vi "Advanced file handeling.vi"(4 "Data in":T1) -> (1 "File out":T2)   [LabVIEW 2014]
uses:
  <vilib>/Utility/file.llb/Read From Spreadsheet File (DBL).vi
panel:
  out "Delimit":string
  in  "File delimit":u16(ring) items=["Tab", "Comma"]
  out "transposed array":dbl[][](array[numeric])
  in  "Test":bool
  in  "Filename No' format":u16(ring) items=["glucose cuvette (#) 0mm.txt", "glucose cuvette (1) #mm.txt"]
  in  "File okay":bool
  in  "Data layout":u16(ring)=1
  out "Modified scan":string[][](table)
  in  "Crop top":i32 min=0
  out "Scan":string[][](table)
  in  "Crop bottom":dbl min=0.0 format="%#.0g"
  in  "Important thing L":i32[](array[numeric])
  in  "Important thing R":i32[](array[numeric])
  in  "Cancel":bool
  in  "OK":bool
  in  "File style":enum32{"Radio Selection 1", "Radio Selection 2"}(radio)
  in  "Select file":bool
  in  "Path":path
  # "Advanced file handling"
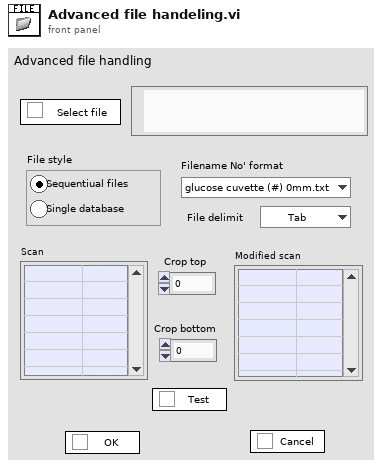
[diagram p1: front panel]
types:
  T1 = cluster{"Path":path, "File style":enum32{"Radio Selection 1", "Radio Selection 2"}, "Filename No' format ":u16, "Data layout":u16, "Crop top":i32, "Crop bottom":dbl, "Important thing R":i32[], "Important thing L":i32[], sgl[][], "Delimit":string}
  T2 = cluster{"Path":path, "File style":enum32{"Radio Selection 1", "Radio Selection 2"}, "Filename No' format ":u16, "Data layout":u16, "Crop top":i32, "Crop bottom":dbl, "Important thing R":i32[], "Important thing L":i32[], sgl[][], "Delimit ":string}
  T3 = enum8{"Enabled", "Disabled", "Disabled and Grayed Out"}
  T4 = cluster{"Path":path, "File style":enum32{"Radio Selection 1", "Radio Selection 2"}, "Filename No' format ":u16, "Data layout":u16, "Crop top":i32, "Crop bottom":dbl, "Important thing R":i32[], "Important thing L":i32[], "transposed array":dbl[][], "Delimit":string}
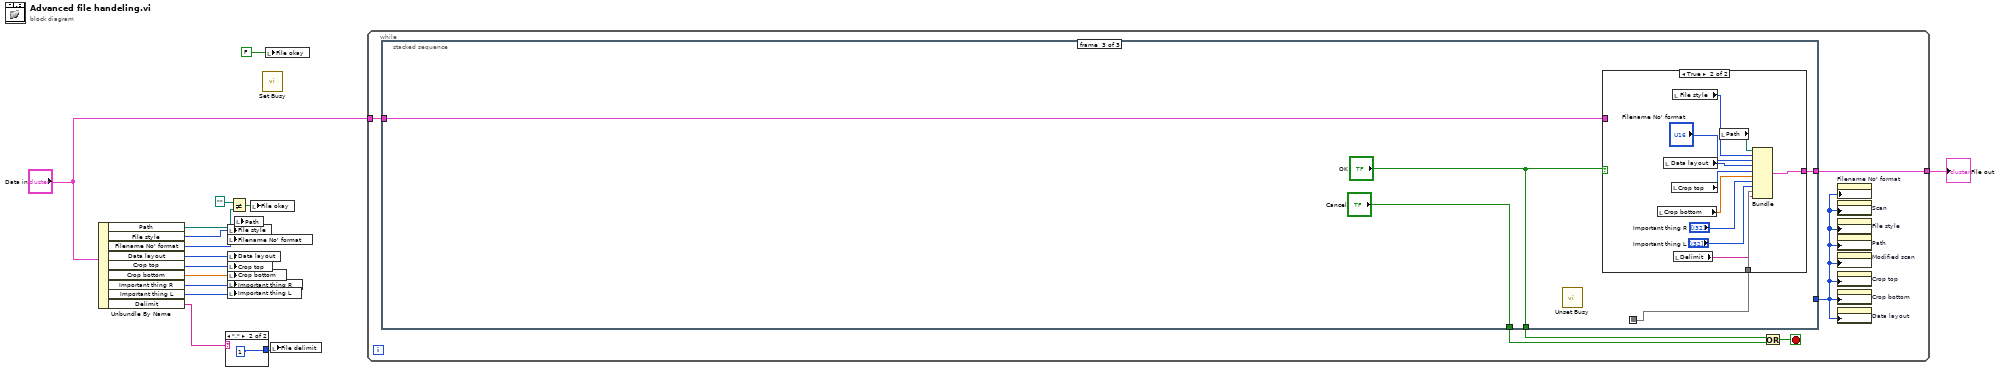
[diagram p0: block diagram]
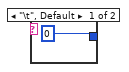
[diagram p2: hidden frame]
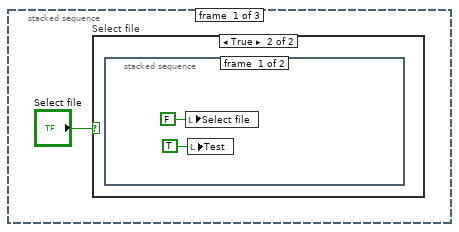
[diagram p3: hidden frame]
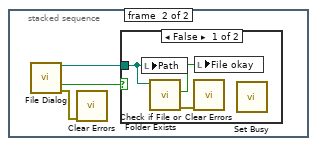
[diagram p5: hidden frame]
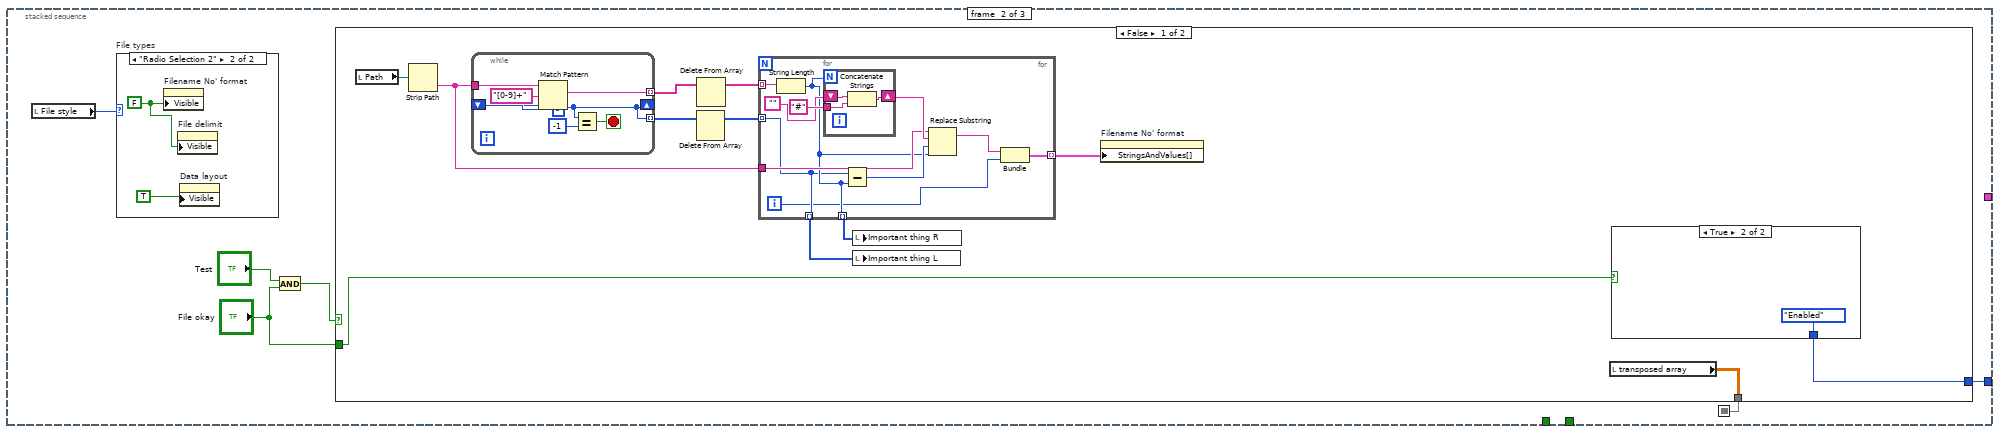
[diagram p7: hidden frame]
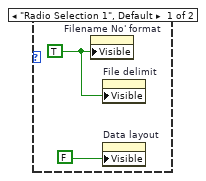
[diagram p8: hidden frame]
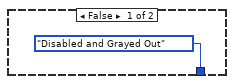
[diagram p9: hidden frame]
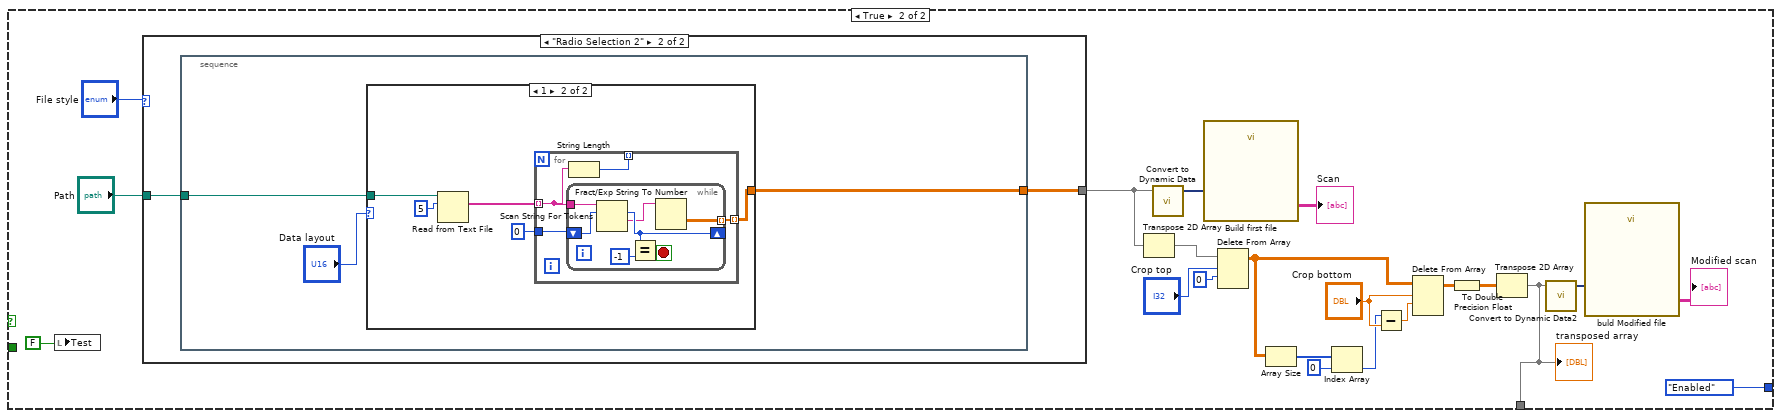
[diagram p10: hidden frame]
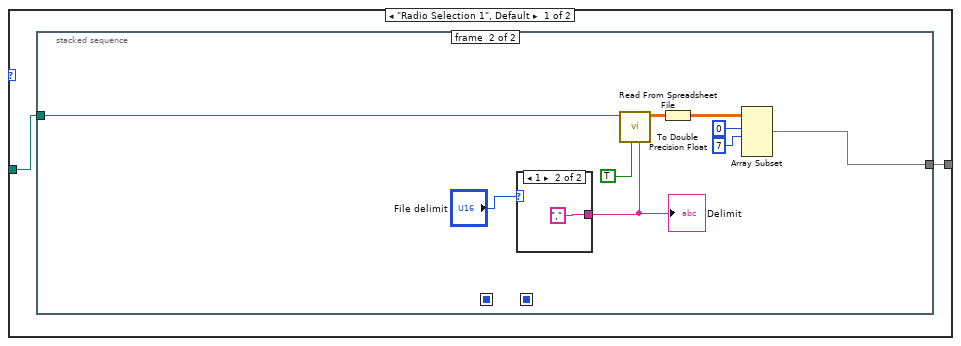
[diagram p11: hidden frame]
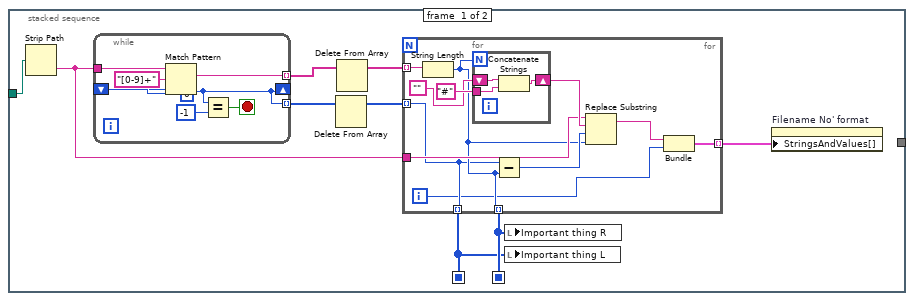
[diagram p12: hidden frame]
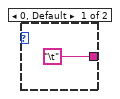
[diagram p13: hidden frame]
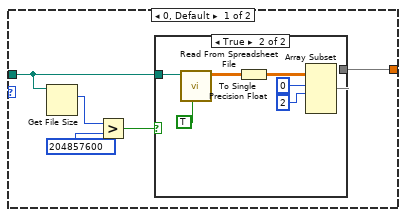
[diagram p14: hidden frame]
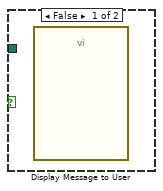
[diagram p15: hidden frame]
diagram:
  n1 = Unbundle By Name("Data in") -> ("Path"=w5:path, "File style"=w11:enum32{"Radio Selection 1", "Radio Selection 2"}, "Filename No' format"=w12:u16, "Data layout"=w10:u16, "Crop top"=w9:i32, "Crop bottom"=w8:dbl, "Important thing R"=w7:i32[], "Important thing L"=w6:i32[], "Delimit"=w2:string)
  n2 = case shown="\",\"" w2 {
    tunnel: [0 1] -> w1
    frame "\t", Default {
    }
    frame "," {
    }
  }
  n3 = local write "File style"(w11) -> ()
  n4 = local write "Filename No' format"(w12) -> ()
  n5 = local write "Data layout"(w10) -> ()
  n6 = local write "Crop top"(w9) -> ()
  n7 = local write "Crop bottom"(w8) -> ()
  n8 = local write "Important thing R"(w7) -> ()
  n9 = local write "Important thing L"(w6) -> ()
  n10 = Not Equal?(x=path "", y=w5) -> (x != y?=w3:bool)
  n11 = local write "Path"(w5) -> ()
  n12 = local write "File okay"(w3) -> ()
  n13 = call <vilib>:"Set Busy.vi"() -> ()  [unwired: 10 in, 2 out]
  n14 = local write "File okay"(FALSE) -> ()
  n15 = local write "File delimit"(w1) -> ()
  n16 = while {
    tunnel: [w20] -> w14
    tunnel: "Data in" -> [w19]
    stop <- w23 stop-if-true
    n17 = stacked-sequence {
      seq-local: [_ w38 _] -> [_ _ w181]
      tunnel: [_ _ "Cancel"] -> w22
      tunnel: [_ _ "OK"] -> w21
      tunnel: [_ _ w178] -> w20
      tunnel: w19 -> [_ _ w177]
      tunnel: [_ w37 _] -> w18
      frame #0 {
        n18 = case "Select file" shown="True" "Select file" {
          frame False {
          }
          frame True {
            n19 = stacked-sequence {
              frame #0 {
                n20 = local write "Select file"(FALSE) -> ()
                n21 = local write "Test"(TRUE) -> ()
              }
              frame #1 {
                n22 = call "File Dialog"() -> ("selected path"=w28:path, "cancelled"=w27:bool, "error out"=w29:errorcluster)  [unwired: 12 in, 1 out]
                n23 = call <vilib>:"Clear Errors.vi"("error in (no error)"=w29) -> ()  [unwired: 5 in, 2 out]
                n24 = case shown="False" w27 {
                  tunnel: w28 -> [w32 _]
                  frame False {
                    n25 = local write "Path"(w32) -> ()
                    n26 = call <vilib>:"Check if File or Folder Exists.vi"("path"=w32) -> ("error out"=w31:errorcluster, "file or folder exists?"=w30:bool)  [unwired: 8 in, 1 out]
                    n27 = call <vilib>:"Clear Errors.vi"("error in (no error)"=w31) -> ()  [unwired: 5 in, 2 out]
                    n28 = local write "File okay"(w30) -> ()
                    n29 = call <vilib>:"Set Busy.vi"() -> ()  [unwired: 10 in, 2 out]
                  }
                  frame True {
                  }
                }
              }
            }
          }
        }
      }
      frame #1 {
        n30 = local read "File style"() -> (w33:enum32{"Radio Selection 1", "Radio Selection 2"})
        n31 = case "File types" shown="\"Radio Selection 2\"" w33 {
          frame "Radio Selection 1", Default {
            w39 = TRUE
            n32 = property on="Filename No' format" class="Ring (strict)"("Visible"=w39) -> ()  [unwired: 2 in, 2 out]
            n33 = property on="File delimit" class="Ring (strict)"("Visible"=w39) -> ()  [unwired: 2 in, 2 out]
            n34 = property on="Data layout" class="Ring (strict)"("Visible"=FALSE) -> ()  [unwired: 2 in, 2 out]
          }
          frame "Radio Selection 2" {
            w41 = FALSE
            n35 = property on="Filename No' format" class="Ring (strict)"("Visible"=w41) -> ()  [unwired: 2 in, 2 out]
            n36 = property on="File delimit" class="Ring (strict)"("Visible"=w41) -> ()  [unwired: 2 in, 2 out]
            n37 = property on="Data layout" class="Ring (strict)"("Visible"=TRUE) -> ()  [unwired: 2 in, 2 out]
          }
        }
        n38 = And(x="Test", y="File okay") -> (x .and. y?=w35:bool)
        n39 = case shown="False" w35 {
          tunnel: [w53 w82] -> w38
          tunnel: [w55 T3."Enabled" ("Disabled")] -> w37
          tunnel: "File okay" -> [w54 _]
          frame False {
            n40 = local read "Path"() -> (w43:path)
            n41 = Strip Path(path=w43) -> (name=w47:string)  [unwired: 1 out]
            n42 = while {
              tunnel: w47 -> [w75]
              shift-right: [w70] -> _
              shift-left: 0 -> [w76]
              tunnel: [w71] -> w50 mode=indexing
              tunnel: [w70] -> w49 mode=indexing
              stop <- w72 stop-if-true
              n43 = Match Pattern(string=w75, regular expression="[0-9]+", offset (0)=w76) -> (match substring=w71:string, offset past match=w70:i32)  [unwired: 2 out]
              n44 = Equal?(x=w70, y=-1) -> (x = y?=w72:bool)
            }
            n45 = Delete From Array(array=w49) -> (array with subset deleted=w52:i32[])  [unwired: 2 in, 1 out]
            n46 = Delete From Array(array=w50) -> (array with subset deleted=w51:string[])  [unwired: 2 in, 1 out]
            n47 = for {
              tunnel: w51 -> [w66] mode=indexing
              tunnel: w52 -> [w57] mode=indexing
              tunnel: [w64] -> w44 mode=indexing
              tunnel: w47 -> [w61]
              tunnel: [w58] -> w46 mode=indexing
              tunnel: [w57] -> w45 mode=indexing
              i -> [w56]
              n48 = String Length(string=w66) -> (length=w58:i32)
              n49 = for {
                N: w58 -> [_]
                shift-right: [w68] -> w62
                shift-left: "" -> [w69]
                tunnel: "#" -> [w67]
                n50 = Concatenate Strings(w69, w67) -> (w68:string)
              }
              n51 = Subtract(x=w57, y=w58) -> (x-y=w59:i32)
              n52 = Replace Substring(2:w58, 3:w59, 4:w62, 5:w61) -> (1:w60:string)  [unwired: 1 out]
              n53 = Bundle("result string"=w60, w56) -> (w64:cluster{"result string":string, i32})  [unwired: 1 in]
            }
            n54 = local write "Important thing R"(w46) -> ()
            n55 = local write "Important thing L"(w45) -> ()
            n56 = property on="Filename No' format" class="Ring (strict)"("StringsAndValues[]"=w44) -> ()  [unwired: 2 in, 2 out]
            n57 = local read "transposed array"() -> (w53:dbl[][])
            n58 = case shown="True" w54 {
              tunnel: [T3."Disabled and Grayed Out" ("Disabled") T3."Enabled" ("Disabled")] -> w55
              frame False {
              }
              frame True {
              }
            }
          }
          frame True {
            n59 = local write "Test"(FALSE) -> ()
            n60 = case shown="\"Radio Selection 2\"" "File style" {
              tunnel: [w101 w145] -> w79
              tunnel: "Path" -> [w100 w144]
              frame "Radio Selection 1", Default {
                n61 = stacked-sequence {
                  seq-local: [w102 _] -> [_ _]
                  seq-local: [w103 _] -> [_ _]
                  tunnel: w100 -> [w106 w133]
                  tunnel: [_ w136] -> w101
                  frame #0 {
                    n62 = Strip Path(path=w106) -> (name=w105:string)  [unwired: 1 out]
                    n63 = while {
                      tunnel: w105 -> [w131]
                      shift-right: [w126] -> _
                      shift-left: 0 -> [w132]
                      tunnel: [w127] -> w109 mode=indexing
                      tunnel: [w126] -> w108 mode=indexing
                      stop <- w128 stop-if-true
                      n64 = Match Pattern(string=w131, regular expression="[0-9]+", offset (0)=w132) -> (match substring=w127:string, offset past match=w126:i32)  [unwired: 2 out]
                      n65 = Equal?(x=w126, y=-1) -> (x = y?=w128:bool)
                    }
                    n66 = Delete From Array(array=w108) -> (array with subset deleted=w111:i32[])  [unwired: 2 in, 1 out]
                    n67 = Delete From Array(array=w109) -> (array with subset deleted=w110:string[])  [unwired: 2 in, 1 out]
                    n68 = for {
                      tunnel: w110 -> [w122] mode=indexing
                      tunnel: w111 -> [w113] mode=indexing
                      tunnel: [w120] -> w104 mode=indexing
                      tunnel: w105 -> [w117]
                      tunnel: [w114] -> w103 mode=indexing
                      tunnel: [w113] -> w102 mode=indexing
                      i -> [w112]
                      n69 = String Length(string=w122) -> (length=w114:i32)
                      n70 = for {
                        N: w114 -> [_]
                        shift-right: [w124] -> w118
                        shift-left: "" -> [w125]
                        tunnel: "#" -> [w123]
                        n71 = Concatenate Strings(w125, w123) -> (w124:string)
                      }
                      n72 = Subtract(x=w113, y=w114) -> (x-y=w115:i32)
                      n73 = Replace Substring(2:w114, 3:w115, 4:w118, 5:w117) -> (1:w116:string)  [unwired: 1 out]
                      n74 = Bundle("result string"=w116, w112) -> (w120:cluster{"result string":string, i32})  [unwired: 1 in]
                    }
                    n75 = local write "Important thing R"(w103) -> ()
                    n76 = local write "Important thing L"(w102) -> ()
                    n77 = property on="Filename No' format" class="Ring (strict)"("StringsAndValues[]"=w104) -> ()  [unwired: 2 in, 2 out]
                  }
                  frame #1 {
                    n78 = case shown="1" "File delimit" {
                      tunnel: ["\t" ("delimiter (\\t)") ","] -> w134
                      frame 0, Default {
                      }
                      frame 1 {
                      }
                    }
                    "Delimit" <- w134
                    n79 = call-poly <vilib>:"Read From Spreadsheet File.vi"("delimiter (\\t)"=w134, "transpose (no:F)"=TRUE, "file path (dialog if empty)"=w133) -> ("all rows"=w141:dbl[][])  [unwired: 4 in, 4 out]
                    n80 = To Double Precision Float(number=w141) -> (double precision float=w137:dbl[][])
                    n81 = Array Subset(array=w137, index (row)=0, length (row)=7) -> (w136:dbl[][])  [unwired: 2 in]
                  }
                }
              }
              frame "Radio Selection 2" {
                n82 = stacked-sequence {
                  tunnel: w144 -> [w147]
                  tunnel: [w148] -> w145
                  frame #0 {
                    n83 = case shown="1" "Data layout" {
                      tunnel: [w153 w161] -> w148
                      tunnel: w147 -> [w151 w164]
                      frame 0, Default {
                        n84 = Get File Size(file=w151) -> (size (in bytes)=w150:i64)  [unwired: 1 in, 2 out]
                        n85 = Greater?(x=w150, y=204857600) -> (0:w149:bool)
                        n86 = case shown="True" w149 {
                          tunnel: [_ w156] -> w153
                          tunnel: w151 -> [_ w154]
                          frame False {
                            n87 = call "Display Message to User"() -> ()  [unwired: 10 in, 2 out]
                          }
                          frame True {
                            n88 = call-poly <vilib>:"Read From Spreadsheet File.vi"("transpose (no:F)"=TRUE, "file path (dialog if empty)"=w154) -> ("all rows"=w160:dbl[][])  [unwired: 5 in, 4 out]
                            n89 = To Single Precision Float(number=w160) -> (single precision float=w159:sgl[][])
                            n90 = Array Subset(array=w159, index (row)=0, length (row)=2) -> (w156:sgl[][])  [unwired: 2 in]
                          }
                        }
                      }
                      frame 1 {
                        n91 = Read from Text File(file (use dialog)=w164, count=5) -> (text=w162:string[])  [unwired: 2 in, 3 out]
                        n92 = for {
                          tunnel: [w169] -> w161 mode=indexing
                          tunnel: 0 -> [w168]
                          tunnel: w162 -> [w167] mode=indexing
                          tunnel: [w166] -> _ mode=indexing
                          n93 = while {
                            tunnel: [w170] -> w169 mode=indexing
                            shift-right: [w175] -> _
                            shift-left: w168 -> [w176]
                            tunnel: w167 -> [w173]
                            stop <- w174 stop-if-true
                            n94 = Scan String For Tokens(8:w176, 9:w173) -> (1:w171:string, 2:w175:i32)  [unwired: 4 in, 2 out]
                            n95 = Equal?(x=w175, y=-1) -> (x = y?=w174:bool)
                            n96 = Fract/Exp String To Number(string=w171) -> (number=w170:dbl)  [unwired: 3 in, 1 out]
                          }
                          n97 = String Length(string=w167) -> (length=w166:i32)
                        }
                      }
                    }
                  }
                }
              }
            }
            n98 = Transpose 2D Array(2D array=w79) -> (transposed array=w84:dbl[][])
            n99 = call "Convert to Dynamic Data"("2D Array"=w79) -> ("Dynamic Data Type"=w98:dynamicdata)  [unwired: 3 in]
            n100 = call "Build first file"("Signals"=w98) -> ("Table"=→"Scan":string[][])  [unwired: 9 in, 1 out]
            n101 = Delete From Array(array=w84, length="Crop top", index (row)=0) -> (array with subset deleted=w96:dbl[][])  [unwired: 1 in, 1 out]
            n102 = Array Size(array=w96) -> (size(s)=w90:i32[])
            n103 = Index Array(array=w90, index=0) -> (element=w93:i32)
            n104 = Subtract(x=w93, y="Crop bottom") -> (x-y=w92:dbl)
            n105 = Delete From Array(array=w96, length="Crop bottom", index (row)=w92) -> (array with subset deleted=w95:dbl[][])  [unwired: 1 in, 1 out]
            n106 = To Double Precision Float(number=w95) -> (double precision float=w83:dbl[][])
            n107 = Transpose 2D Array(2D array=w83) -> (transposed array=w82:dbl[][])
            "transposed array" <- w82
            n108 = call "Convert to Dynamic Data2"("2D Array"=w82) -> ("Dynamic Data Type"=w87:dynamicdata)  [unwired: 3 in]
            n109 = call "buld Modified file"("Signals"=w87) -> ("Table"=→"Modified scan":string[][])  [unwired: 9 in, 1 out]
          }
        }
      }
      frame #2 {
        n110 = call <vilib>:"Unset Busy.vi"() -> ()  [unwired: 11 in, 1 out]
        n111 = case shown="True" "OK" {
          tunnel: w181 -> [_ w185]
          tunnel: [w182 w184] -> w178
          tunnel: w177 -> [w182 _]
          frame False {
          }
          frame True {
            n112 = local read "Crop bottom"() -> (w188:dbl)
            n113 = local read "Data layout"() -> (w190:u16)
            n114 = local read "Crop top"() -> (w189:i32)
            n115 = local read "File style"() -> (w192:enum32{"Radio Selection 1", "Radio Selection 2"})
            n116 = local read "Delimit"() -> (w183:string)
            n117 = local read "Path"() -> (w193:path)
            n118 = Bundle("Path"=w193, "File style"=w192, "Filename No' format"="Filename No' format", "Data layout"=w190, "Crop top"=w189, "Crop bottom"=w188, "Important thing R"="Important thing R", "Important thing L"="Important thing L", "transposed array"=w185, "Delimit"=w183) -> (w184:T4)  [unwired: 1 in]
          }
        }
      }
    }
    n119 = Or(x=w21, y=w22) -> (x .or. y?=w23:bool)
    n120 = property on="Scan" class="Tbl (strict)"("DisabledEnum"=w18) -> ()  [unwired: 2 in, 2 out]
    n121 = property on="File style" class="RadioBtnsControl (strict)"("DisabledEnum"=w18) -> ()  [unwired: 2 in, 2 out]
    n122 = property on="Path" class="Path"("DisabledEnum"=w18) -> ()  [unwired: 2 in, 2 out]
    n123 = property on="Modified scan" class="Tbl (strict)"("DisabledEnum"=w18) -> ()  [unwired: 2 in, 2 out]
    n124 = property on="Crop top" class="DigNum (strict)"("DisabledEnum"=w18) -> ()  [unwired: 2 in, 2 out]
    n125 = property on="Crop bottom" class="DigNum (strict)"("DisabledEnum"=w18) -> ()  [unwired: 2 in, 2 out]
    n126 = property on="Data layout" class="Ring (strict)"("DisabledEnum"=w18) -> ()  [unwired: 2 in, 2 out]
    n127 = property on="Filename No' format" class="Ring (strict)"("DisabledEnum"=w18) -> ()  [unwired: 2 in, 2 out]
  }
  "File out" <- w14
